vi "Valve Close.vi"(8 "error in (no error)":errorcluster, 11 "DAC Vacum Valve in":refnum<class "DAC Vacum Valve.lvclass">) -> (0 "error out":errorcluster, 3 "DAC Vacum Valve out":refnum<class "DAC Vacum Valve.lvclass">)   [LabVIEW 2019, in "DAC.lvlib" / "DAC Vacum Valve.lvclass"]
uses:
  DAC Vacum Valve.lvclass
  DAC Vacum Valve.lvclass/DAC Vacum Valve.ctl
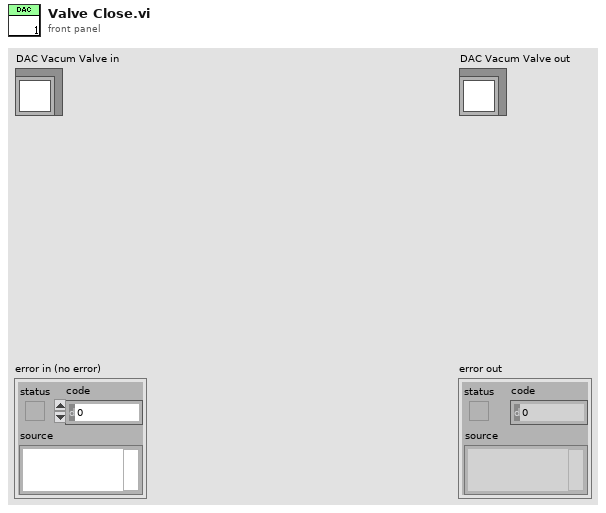
[diagram p1: front panel]
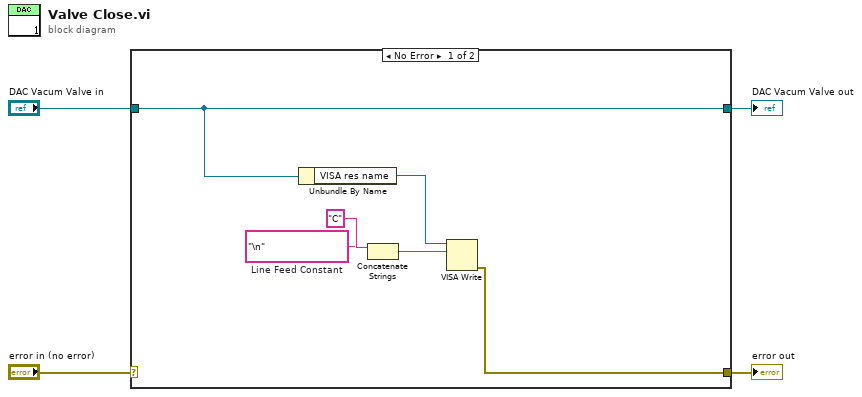
[diagram p0: block diagram]
diagram:
  n1 = case shown="No Error" "error in (no error)" {
    selector: "error in (no error)" -> [_ w12]
    tunnel: [w5 w12] -> w3
    tunnel: [w10 w11] -> w1
    tunnel: "DAC Vacum Valve in" -> [w10 w11]
    frame No Error {
      w7 = "\n"  # Line Feed Constant
      n2 = Unbundle By Name(w10) -> ("VISA res name"=w9:refnum<visa-resource-name>)
      n3 = Concatenate Strings("C" ("string"), w7) -> (w6:string)
      n4 = VISA Write(VISA resource name=w9, write buffer=w6) -> (error out=w5:errorcluster)  [unwired: 1 in, 2 out]
    }
    frame Error {
    }
  }
  "error out" <- w3
  "DAC Vacum Valve out" <- w1
